vi "Open Note File.vi"(8 "Error In":errorcluster, 10 "SR Number":i32, 11 "Folder path":path) -> (0 "Error Out":errorcluster, 2 "Notes":string, 3 "file path":path)   [LabVIEW 2018]
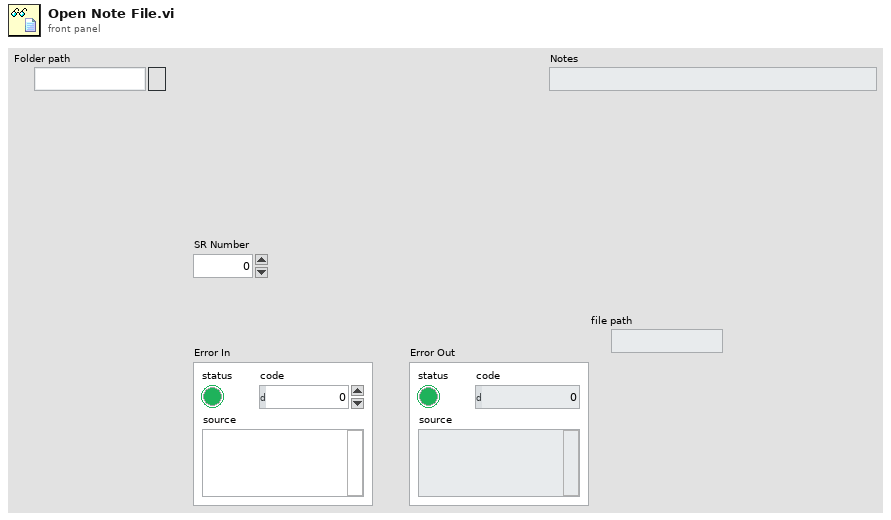
[diagram p1: front panel]
types:
  T1 = enum16{"open", "replace", "create", "open or create", "replace or create", "replace or create with confirmation"}
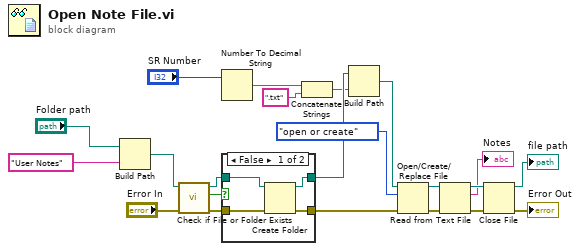
[diagram p0: block diagram]
diagram:
  n1 = Build Path(base path="Folder path", name or relative path="User Notes") -> (appended path=w14:path)
  n2 = call <vilib>:"Check if File or Folder Exists.vi"("error in (no error)"="Error In", "path"=w14) -> ("error out"=w17:errorcluster, "file or folder exists?"=w18:bool, "dup path"=w16:path)  [unwired: 7 in]
  n3 = Number To Decimal String(number="SR Number") -> (decimal integer string=w10:string)  [unwired: 1 in]
  n4 = case shown="False" w18 {
    tunnel: w17 -> [w26 w27]
    tunnel: w16 -> [w25 w28]
    tunnel: [w24 w28] -> w15
    tunnel: [w23 w27] -> w7
    frame False {
      n5 = Create Folder(path (use dialog)=w25, error in=w26) -> (created path=w24:path, error out=w23:errorcluster)  [unwired: 1 in, 1 out]
    }
    frame True {
    }
  }
  n6 = Concatenate Strings(w10, ".txt" ("string")) -> (w8:string)
  n7 = Build Path(base path=w15, name or relative path=w8) -> (appended path=w12:path)
  n8 = Open/Create/Replace File(file path (use dialog)=w12, error in=w7, operation (0:open)=T1."open or create") -> (refnum out=w22:refnum<file>, error out=w21:errorcluster)  [unwired: 3 in, 1 out]
  n9 = Read from Text File(file (use dialog)=w22, error in=w21) -> (refnum out=w20:refnum<file>, text=→"Notes":string, error out=w2:errorcluster)  [unwired: 2 in, 1 out]
  n10 = Close File(refnum=w20, error in=w2) -> (path=→"file path":path, error out=→"Error Out":errorcluster)
